vi "GUI_HTU_EMQ_triplet.vi"() -> ()   [LabVIEW 2020]
uses:
  Shared/GUI_Template/GUI_master/tcp_new_data_event.ctl
  Shared/GUI_Template/GUI_master/tcp new data cluster.ctl
panel:
  in  "abort3":bool
  in  "abort2":bool
  out "Chart":cluster{dbl, dbl, dbl}(graph)
  in  "Degauss max\ncurrent":dbl=1.0
  in  "EMQ3":bool
  in  "EMQ2":bool
  out "EMQ3 indicator":bool
  out "EMQ2 indicator":bool
  out "EMQ1 indicator":bool
  in  "EMQ1":bool
  in  "abort1":bool
  in  "SwitchWait":dbl=1500.0 min=0.0 max=12.0
  in  "EMQ3Reset":bool caption="Blank Button"
  in  "EMQ3Switch":bool caption="Blank Button"
  in  "EMQ2Reset":bool caption="Blank Button"
  in  "EMQ2Switch":bool caption="Blank Button"
  in  "EMQ1Reset":bool caption="Blank Button"
  in  "EMQ1Switch":bool caption="Blank Button"
  in  "DigitalOutput.Channel 4::4":bool=TRUE caption="Blank Button"
  in  "DigitalOutput.Channel 5::4":bool=TRUE caption="Blank Button"
  in  "DigitalOutput.Channel 2::4":bool=TRUE caption="Blank Button"
  in  "DigitalOutput.Channel 3::4":bool=TRUE caption="Blank Button"
  out "XY Graph":cluster{dbl[], dbl[]}(graph)
  in  "CurrentSwitch limit":dbl=0.03 min=0.0 max=12.0
  in  "GUIdevice 4":string="U_SSR_2"
  out "Power.Ch2::1":dbl caption="Power::2" min=0.0 max=12.0
  out "Voltage.Ch2::1":dbl caption="Voltage::2" min=0.0 max=12.0
  out "Current.Ch2::1":dbl caption="Current::2" min=0.0 max=12.0
  out "Power.Ch3::1":dbl caption="Power::3" min=0.0 max=12.0
  out "Voltage.Ch3::1":dbl caption="Voltage::3" min=0.0 max=12.0
  out "Current.Ch3::1":dbl caption="Current::3" min=0.0 max=12.0
  out "Power.Ch1::1":dbl caption="Power::1" min=0.0 max=12.0
  out "Voltage.Ch1::1":dbl caption="Voltage::1" min=0.0 max=12.0
  out "Current.Ch1::1":dbl caption="Current::1" min=0.0 max=12.0
  in  "Voltage_Limit.Ch3::1":dbl caption="EMQ3 Voltage" min=0.0 max=6.0
  in  "Enable_Output.Ch3::1":enum16{"on", "off"}(ring) caption="Enable EMQ3"
  in  "Current_Limit.Ch3::1":dbl caption="EMQ3 Current" min=0.0 max=6.0
  in  "Voltage_Limit.Ch1::1":dbl caption="EMQ1 Voltage" min=0.0 max=6.0
  in  "Voltage_Limit.Ch2::1":dbl caption="EMQ2 Voltage" min=0.0 max=8.0
  in  "Enable_Output.Ch2::1":enum16{"on", "off"}(ring) caption="Enable EMQ2"
  in  "Enable_Output.Ch1::1":enum16{"on", "off"}(ring) caption="Enable EMQ1"
  in  "Current_Limit.Ch1::1":dbl caption="EMQ1 Current" min=0.0 max=6.0
  in  "Current_Limit.Ch2::1":dbl caption="EMQ2 Current" min=0.0 max=6.0
  in  "UDP error message":string
  in  "GUIdevice 1":string="U_EMQTriplet"
  in  "DigitalOutput.Channel 0::4":bool=TRUE caption="Blank Button"
  in  "DigitalOutput.Channel 1::4":bool=TRUE caption="Blank Button"
  out "error IO 2":errorcluster
  out "tcp data event":T1
  in  "stop":bool
  # "HTU EMQ Triplet"
  # "Polarity indicator"
  # "Polarity switch"
  # "Polarity reset"
  # "Degaussing"
  # "EMQ1\nEMQ1"
  # "EMQ2\nEMQ2"
  # "EMQ3"
  # "Enable output"
  # "Current Limit"
  # "Voltage Limit"
  # "Current"
  # "Voltage"
  # "Power"
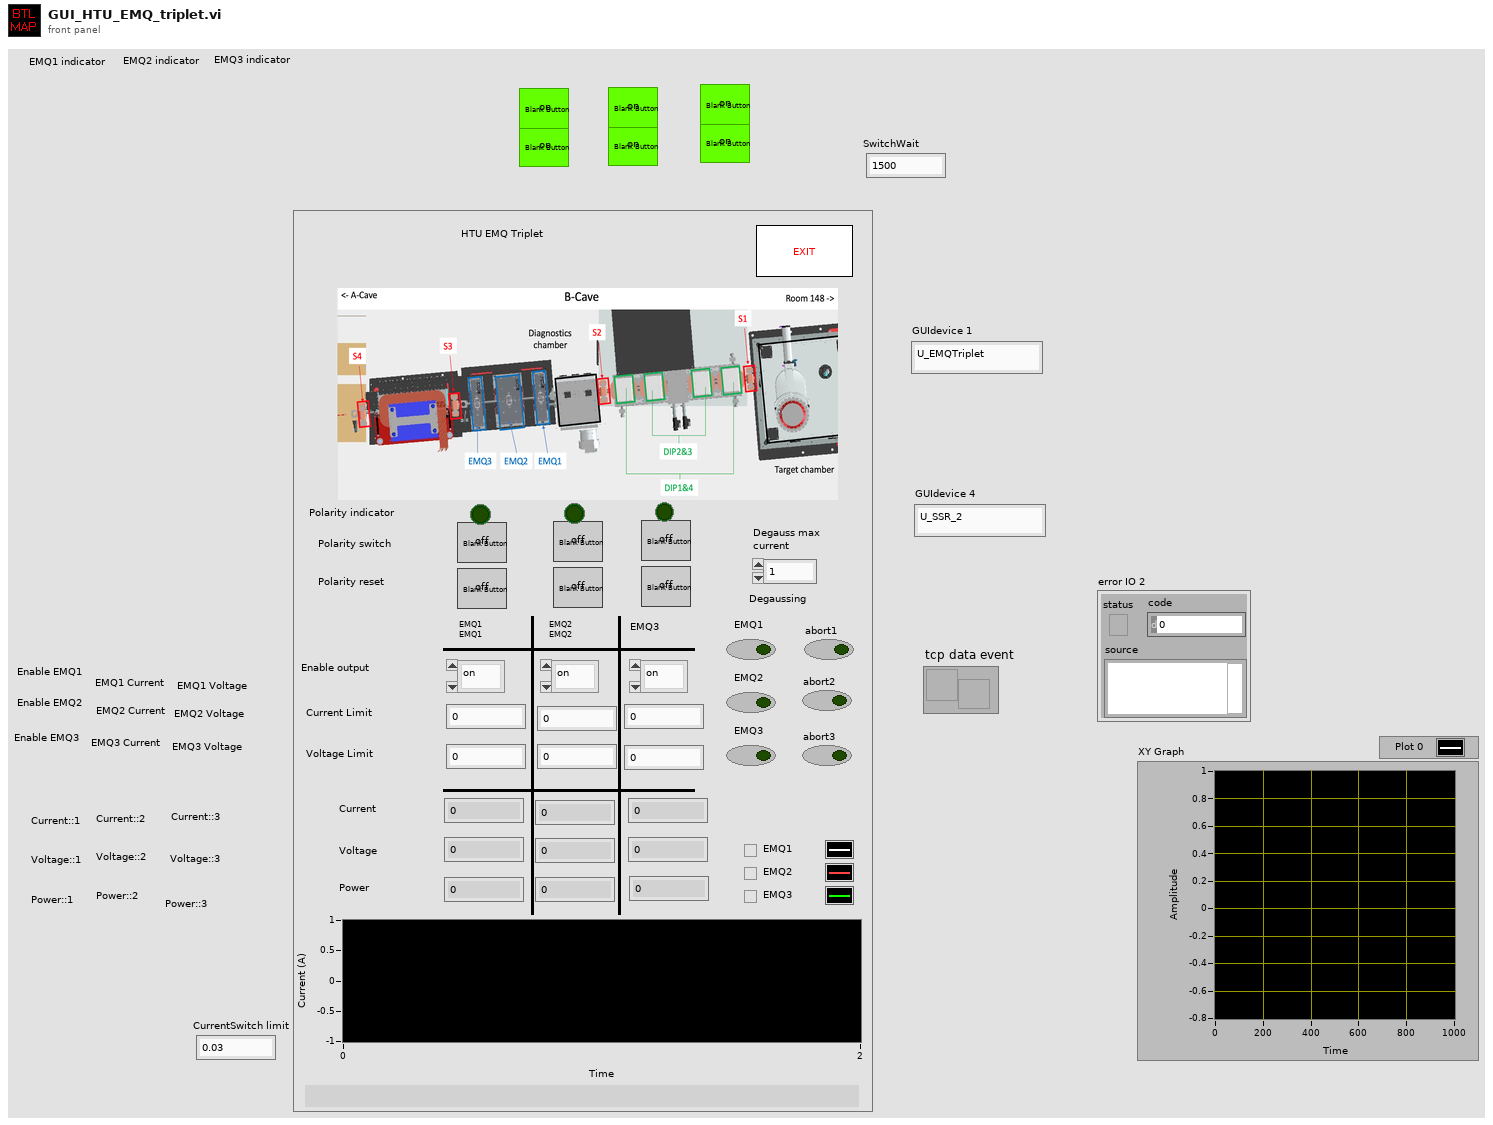
[diagram p1: front panel]
types:
  T1 = typedef "tcp_new_data_event.ctl" = refnum<user-event>
  T2 = typedef "tcp new data cluster.ctl" = cluster{"EventEnum":enum16{"new data", "connection status update"}, "Device name":string}
  T3 = enum32{"invalid app kind", "Development System", "Run Time System", "Student Edition", "Embedded LabVIEW", "Evaluation", "Custom"}
  T4 = enum32{"Invalid", "Standard", "Closed", "Hidden", "Minimized", "Maximized"}
  T5 = cluster{"Core":cluster{"Current VI Reference":refnum<vi>, "Close Panel on Exit?":bool}, "CurrentGraph1":dbl[][], "EMQ1PolaritySwitched":bool, "EMQ2PolaritySwitched":bool, "EMQ3PolaritySwitched":bool, "DegaussEMQ1":bool, "degauss loop":i32, "EMQ1DegaussSetCur":dbl, "EMQ2DegaussSetCur":dbl, "EMQ3DegaussSetCur":dbl, "last chart update tck":i32}
  T6 = cluster{"Current VI Reference":refnum<vi>, "Close Panel on Exit?":bool}
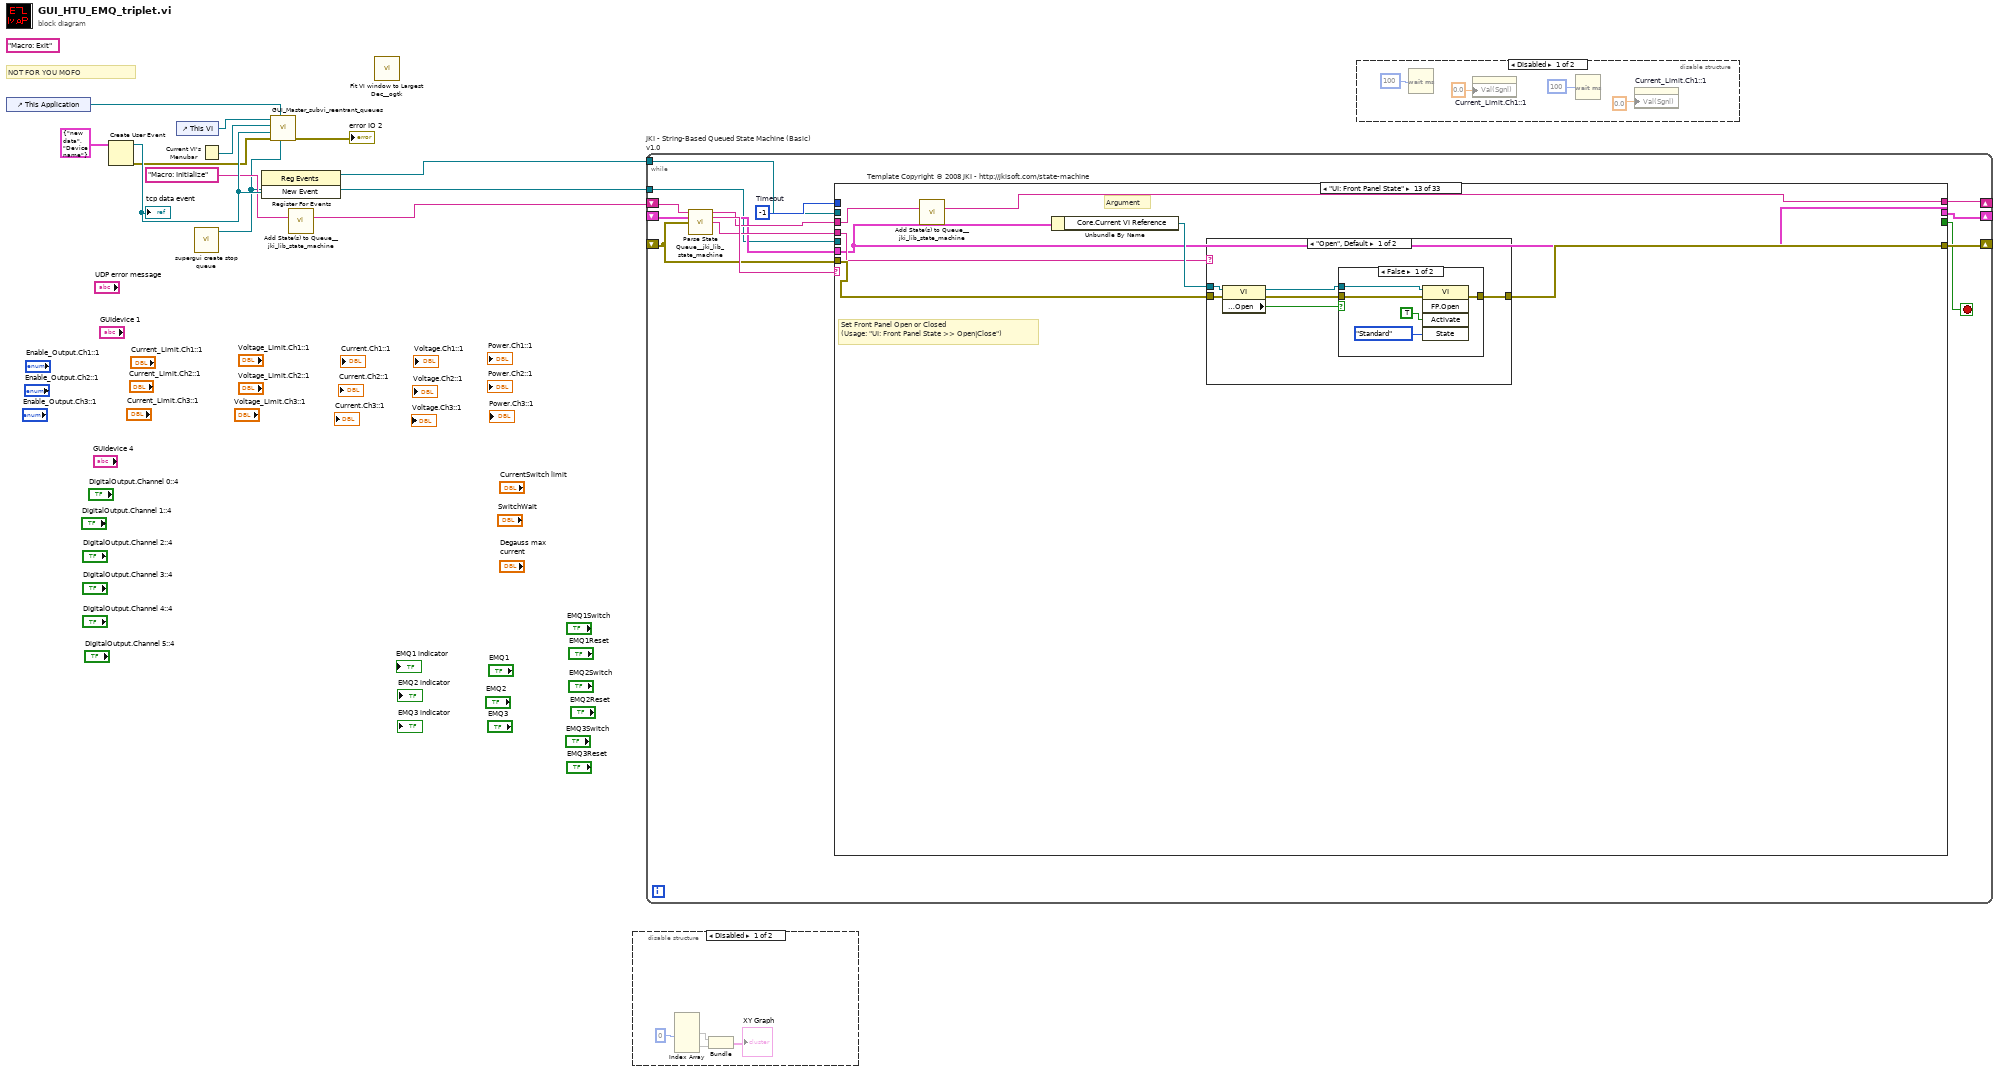
[diagram p0: block diagram]
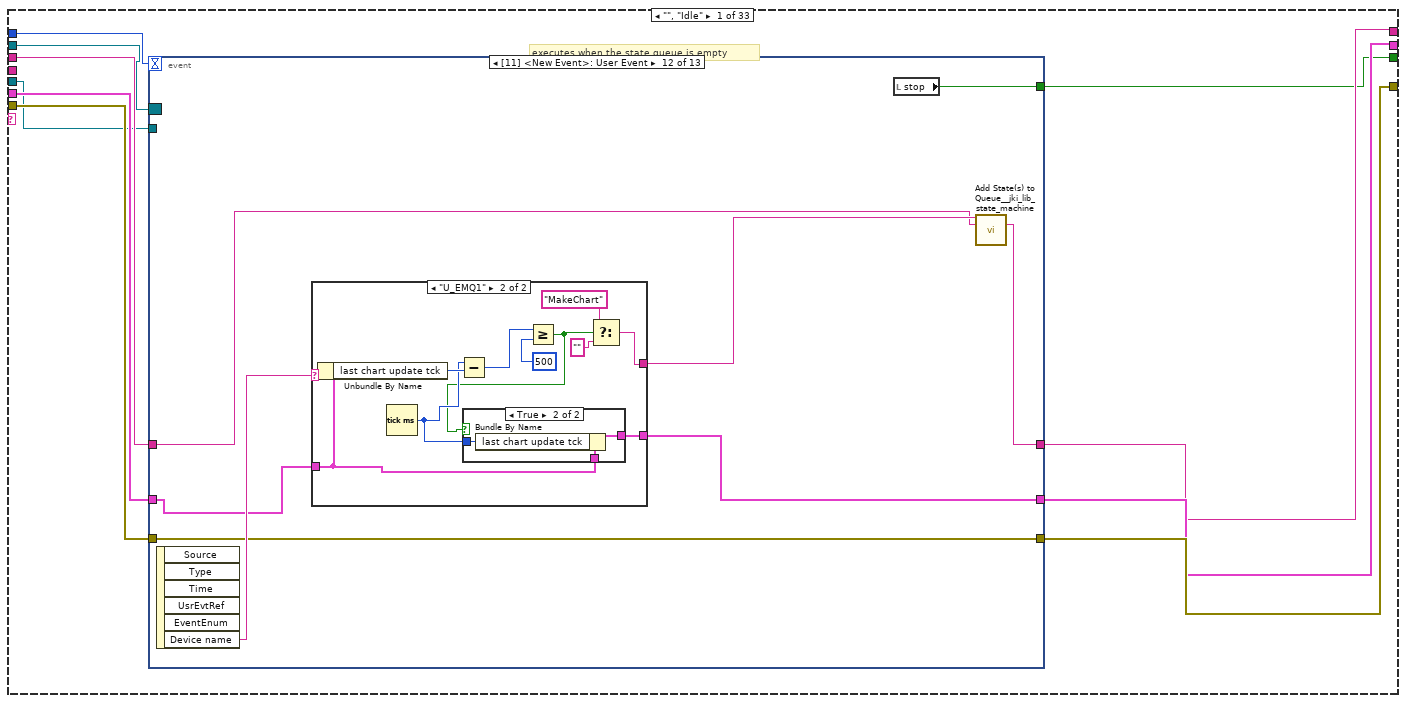
[diagram p4: hidden frame]
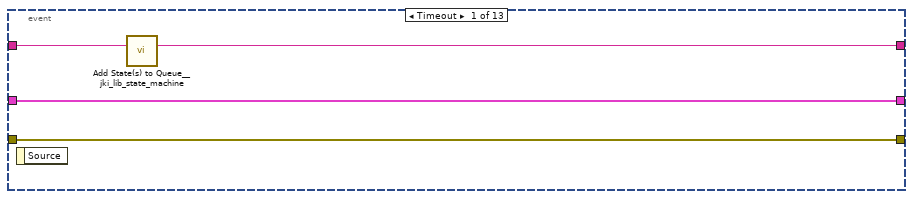
[diagram p5: hidden frame]
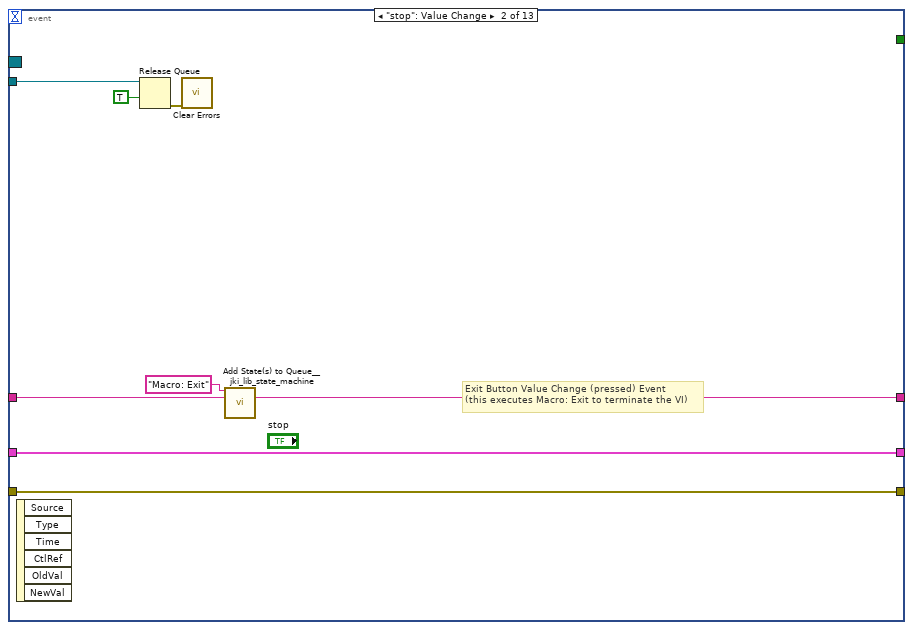
[diagram p6: hidden frame]
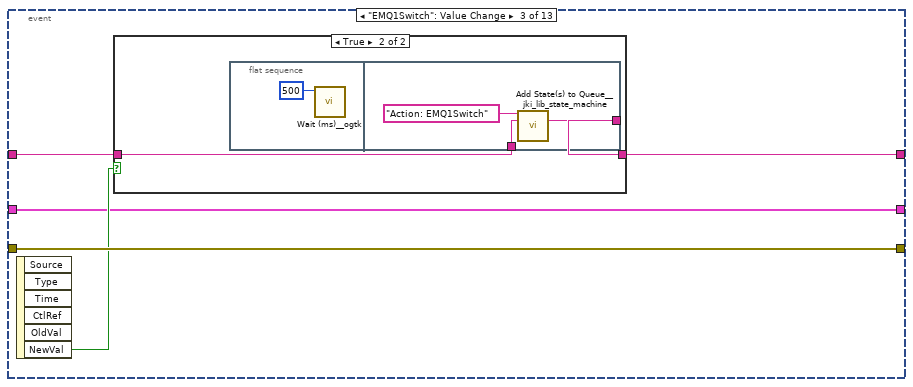
[diagram p7: hidden frame]
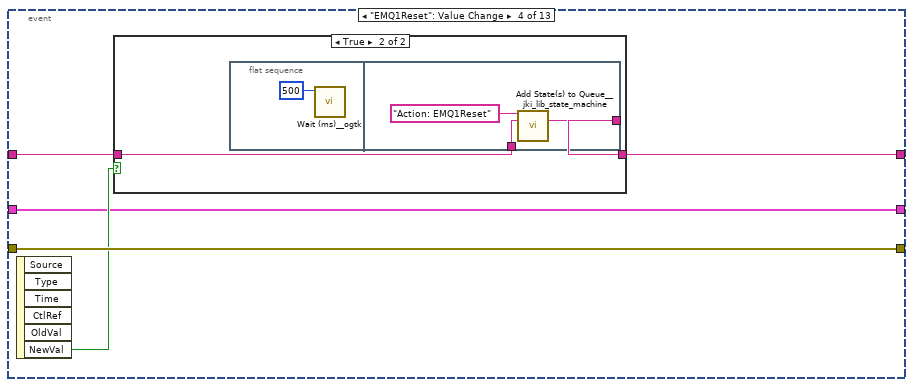
[diagram p9: hidden frame]
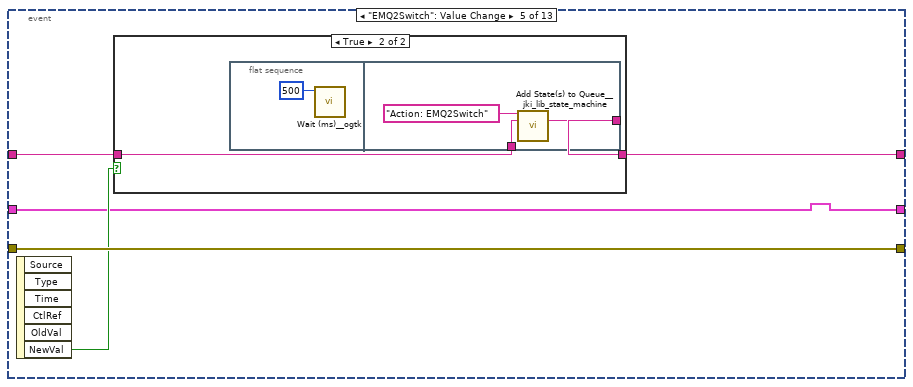
[diagram p11: hidden frame]
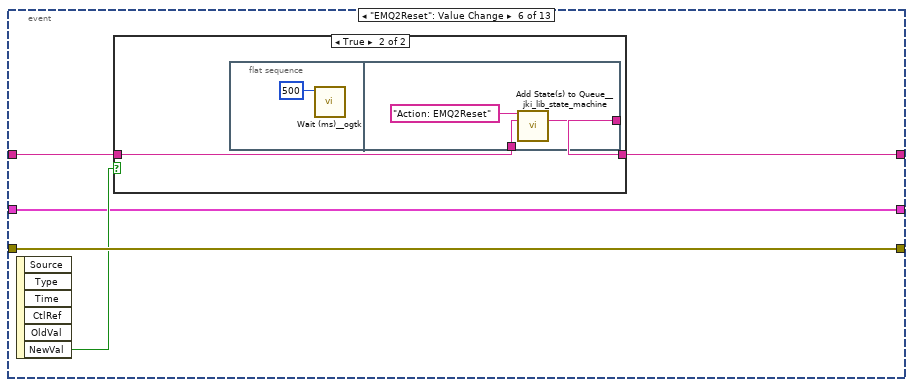
[diagram p13: hidden frame]
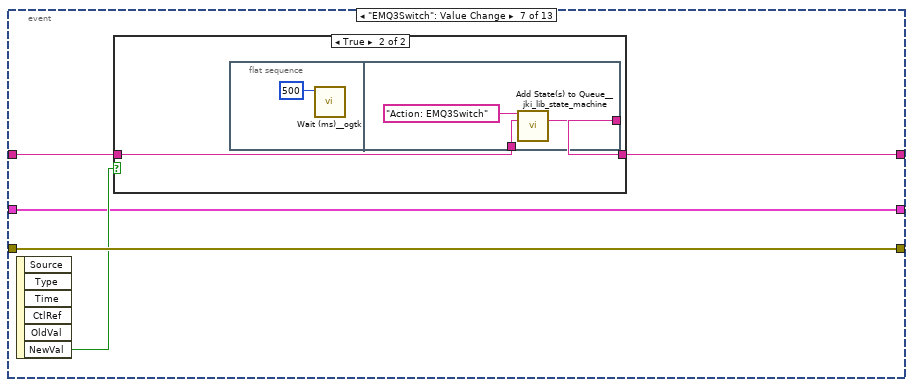
[diagram p15: hidden frame]
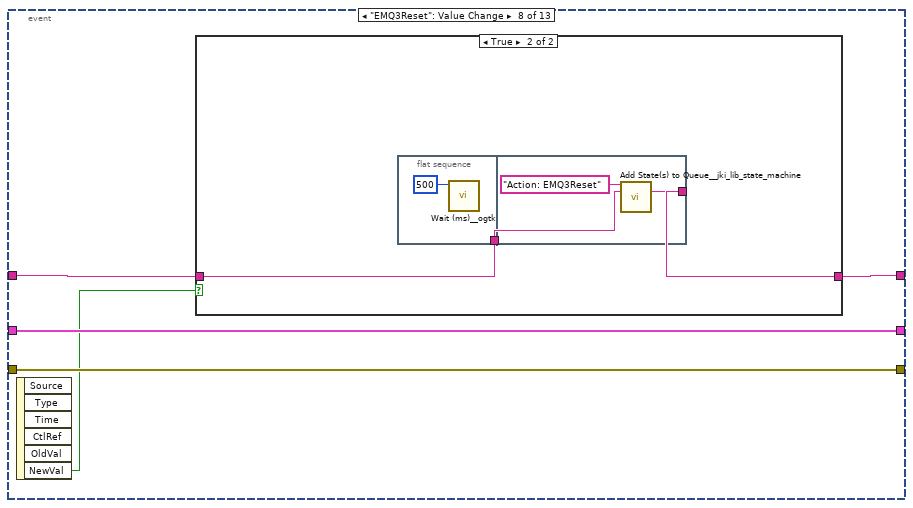
[diagram p17: hidden frame]
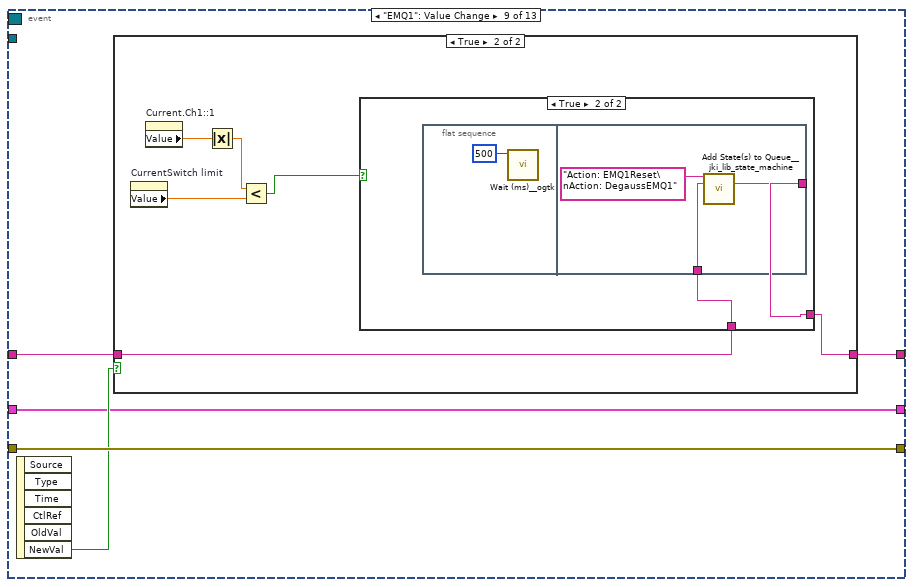
[diagram p19: hidden frame]
diagram:
  (unwired) "Macro: Exit"
  # "NOT FOR YOU MOFO"
  n1 = control-ref of="This Application"() -> (w11:refnum<vi>)
  n2 = Create User Event(user event datatype=T2 {"EventEnum"=enum."new data", "Device name"="Device name"} ("New Event")) -> (user event=w10:refnum<user-event>, error out=w9:errorcluster)  [unwired: 1 in]
  "tcp data event" <- w10
  n3 = control-ref of="This VI"() -> (w5:refnum<vi>)
  n4 = call "supergui create stop queue.vi"() -> ("STOP Queue out"=w1:refnum<queue>)  [unwired: 11 in]
  n5 = Current VI's Menubar() -> (w7:refnum<k9>)
  n6 = register-events(w10) -> (reference out=w2:refnum<event-registration>)  [unwired: 2 in, 1 out]
  n7 = call "GUI_Master_subvi_reentrant_queues.vi"("STOP Queue in"=w1, "This Application"=w11, "error in (no error)"=w9, "tcp data event"=w10, "Caller menu reference"=w7, "Caller VI ref"=w5) -> ("error out"=→"error IO 2":errorcluster)  [unwired: 5 in]
  n8 = call <vilib>:"Add State(s) to Queue__jki_lib_state_machine.vi"("State(s) in (\"\")"="Macro: Initialize") -> ("States Out"=w3:string)  [unwired: 14 in]
  n9 = call <userlib>:"Fit VI window to Largest Dec__ogtk.vi"() -> ()  [unwired: 6 in, 2 out]
  n10 = disable-structure shown="Disabled" {
    frame Disabled {
      n11 = Index Array(index (col) #1=0 ("disabled index (col)")) -> (array=w16:dbl[][], element #1=w12, element #2=w13)  [unwired: 3 in]
      n12 = Bundle(w12, w13) -> (→"XY Graph":cluster{void, void})  [unwired: 1 in]
    }
    frame Enabled {
    }
  }
  n13 = while "JKI - String-Based Queued State Machine (Basic) v1.0" {
    shift-right: [w23] -> _
    shift-left: _ -> [w22]
    shift-right: [w25] -> _
    shift-left: _ -> [w20]
    shift-right: [w17] -> _
    shift-left: w3 -> [w26]
    tunnel: w2 -> [w19]
    tunnel: w1 -> [w18]
    stop <- w24 stop-if-true
    w21 = -1  # Timeout
    # "Template Copyright © 2008 JKI - http://jkisoft.com/state-machine"
    n14 = call <vilib>:"Parse State Queue__jki_lib_state_machine.vi"("State Queue"=w26, "Error In (no error)"=w20) -> ("Remaining States"=w28:string, "Current State"=w29:string, "Arguments"=w27:string)  [unwired: 11 in]
    n15 = case shown="\"UI: Front Panel State\"" w29 {
      selector: w29 -> [_ _ w215 _ _ _ _ _ _ _ _ _ _ _ _ _ _ _ _ _ _ _ _ _ _ _ _ _ _ _ _ _ _]
      tunnel: w28 -> [w39 w213 w218 w236 w242 w247 w251 w266 w272 w276 w280 w286 w297 w323 w328 w338 w342 w352 w375 w398 w421 w444 w467 w486 w496 w506 w517 w585 w653 w716 w733 w749 w777]
      tunnel: w27 -> [_ _ _ _ _ _ _ _ _ _ _ w282 w293 _ _ _ _ _ _ _ _ _ _ _ _ _ _ _ _ _ _ _ _]
      tunnel: w22 -> [w38 w211 w217 w228 w241 w246 w249 _ w268 w274 w279 w285 w292 w321 w326 w330 w340 w346 w369 w392 w415 w436 w459 w484 w494 w504 w518 w586 w654 w720 w736 w752 w767]
      tunnel: [w37 w212 w220 w225 errorcluster {"status"=FALSE, "code"=0, "source"=""} ("error out") w245 w250 w265 w270 w275 w278 w283 w295 w322 w327 w337 w341 w343 w366 w389 w412 w437 w460 w487 w497 w507 w511 w579 w647 w721 w737 w753 w778] -> w25
      tunnel: w20 -> [w36 w212 w219 w225 w240 w245 w250 w265 w271 w275 w278 w284 w296 w322 w327 w337 w341 w344 w367 w390 w413 w438 w461 w487 w497 w507 w512 w580 w648 w721 w737 w753 w778]
      tunnel: [w30 _ _ _ _ TRUE _ _ _ _ _ _ _ _ _ _ _ _ _ _ _ _ _ _ _ _ _ _ _ _ _ _ _] -> w24
      tunnel: [w33 w211 w217 w227 w241 w246 w249 w255 w268 w274 w279 w285 w292 w321 w326 w330 w340 w345 w368 w391 w414 w435 w458 w483 w493 w503 w515 w583 w651 w720 w736 w752 w767] -> w23
      tunnel: w21 -> [w35 _ _ _ _ _ _ _ _ _ _ _ _ _ _ _ _ _ _ _ _ _ _ _ _ _ _ _ _ _ _ _ _]
      tunnel: w19 -> [w31 _ _ _ _ _ _ _ _ _ _ _ _ _ _ _ _ _ _ _ _ _ _ _ _ _ _ _ _ _ _ _ _]
      tunnel: w18 -> [w34 _ _ _ _ _ _ _ _ _ _ _ _ _ _ _ _ _ _ _ _ _ _ _ _ _ _ _ _ _ _ _ _]
      tunnel: [w32 w210 w214 w226 w237 w243 w248 w261 w267 w273 w277 w281 w291 w320 w324 w329 w339 w351 w374 w397 w420 w443 w466 w485 w495 w505 w516 w584 w652 w718 w734 w750 w777] -> w17
      frame "", "Idle" {
        # "executes when the state queue is empty"
        n16 = event shown="[11] <New Event>: User Event" {
          selector: w31 -> [_ _ _ _ _ _ _ _ _ _ _ _ _]
          dyn-events: _ -> [_ _ _ _ _ _ _ _ _ _ _ _ _]
          timeout: w35 -> [_ _ _ _ _ _ _ _ _ _ _ _ _]
          tunnel: w39 -> [w43 w51 w54 w66 w78 w90 w102 w115 w126 w145 w164 w186 w209]
          tunnel: [w42 w50 w53 w65 w77 w89 w101 w114 w125 w144 w163 w185 w208] -> w32
          tunnel: w38 -> [w40 w48 w52 w64 w76 w88 w100 w113 w124 w143 w162 w182 w206]
          tunnel: [w41 w49 w56 w68 w80 w92 w104 w116 w128 w147 w166 w184 w207] -> w37
          tunnel: w36 -> [w41 w49 w56 w68 w80 w92 w104 w116 w128 w147 w166 w184 w207]
          tunnel: [w40 w48 w52 w64 w76 w88 w100 w113 w124 w143 w162 w181 w206] -> w33
          tunnel: w34 -> [_ w45 _ _ _ _ _ _ _ _ _ _ _]
          tunnel: [_ _ _ _ _ _ _ _ _ _ _ w183 _] -> w30
          event Timeout {
            n17 = event-data() -> ()  [unwired: 1 in, 1 out]
            n18 = call <vilib>:"Add State(s) to Queue__jki_lib_state_machine.vi"("State(s) in (\"\")"=w43) -> ("States Out"=w42:string)  [unwired: 14 in]
          }
          event "stop": Value Change {
            # "Exit Button Value Change (pressed) Event\n(this executes Macro: Exit to terminate the VI)"
            n19 = event-data() -> ()  [unwired: 1 in, 6 out]
            n20 = Release Queue(queue=w45, force destroy? (F)=TRUE) -> (error out=w46:errorcluster)  [unwired: 1 in, 2 out]
            n21 = call <vilib>:"Clear Errors.vi"("error in (no error)"=w46) -> ()  [unwired: 5 in, 2 out]
            n22 = call <vilib>:"Add State(s) to Queue__jki_lib_state_machine.vi"("State(s) in Front (\"\")"="Macro: Exit", "State(s) in (\"\")"=w51) -> ("States Out"=w50:string)  [unwired: 13 in]
          }
          event "EMQ1Switch": Value Change {
            n23 = event-data() -> ("NewVal"=w55:bool)  [unwired: 1 in, 5 out]
            n24 = case shown="True" w55 {
              tunnel: w54 -> [w57 w59]
              tunnel: [w57 w58] -> w53
              frame False {
              }
              frame True {
                n25 = flat-sequence {
                  tunnel: w59 -> [w62]
                  tunnel: [w61] -> w58
                  frame #0 {
                    n26 = call <userlib>:"Wait (ms)__ogtk.vi"("milliseconds to wait"=u32 500) -> ()  [unwired: 9 in, 2 out]
                  }
                  frame #1 {
                    n27 = call <vilib>:"Add State(s) to Queue__jki_lib_state_machine.vi"("State(s) in Front (\"\")"="Action: EMQ1Switch" ("State(s) in Front (\"\")"), "State(s) in (\"\")"=w62) -> ("States Out"=w61:string)  [unwired: 13 in]
                  }
                }
              }
            }
          }
          event "EMQ1Reset": Value Change {
            n28 = event-data() -> ("NewVal"=w67:bool)  [unwired: 1 in, 5 out]
            n29 = case shown="True" w67 {
              tunnel: w66 -> [w69 w71]
              tunnel: [w69 w70] -> w65
              frame False {
              }
              frame True {
                n30 = flat-sequence {
                  tunnel: w71 -> [w74]
                  tunnel: [w73] -> w70
                  frame #0 {
                    n31 = call <userlib>:"Wait (ms)__ogtk.vi"("milliseconds to wait"=u32 500) -> ()  [unwired: 9 in, 2 out]
                  }
                  frame #1 {
                    n32 = call <vilib>:"Add State(s) to Queue__jki_lib_state_machine.vi"("State(s) in Front (\"\")"="Action: EMQ1Reset" ("State(s) in Front (\"\")"), "State(s) in (\"\")"=w74) -> ("States Out"=w73:string)  [unwired: 13 in]
                  }
                }
              }
            }
          }
          event "EMQ2Switch": Value Change {
            n33 = event-data() -> ("NewVal"=w79:bool)  [unwired: 1 in, 5 out]
            n34 = case shown="True" w79 {
              tunnel: w78 -> [w81 w83]
              tunnel: [w81 w82] -> w77
              frame False {
              }
              frame True {
                n35 = flat-sequence {
                  tunnel: w83 -> [w86]
                  tunnel: [w85] -> w82
                  frame #0 {
                    n36 = call <userlib>:"Wait (ms)__ogtk.vi"("milliseconds to wait"=u32 500) -> ()  [unwired: 9 in, 2 out]
                  }
                  frame #1 {
                    n37 = call <vilib>:"Add State(s) to Queue__jki_lib_state_machine.vi"("State(s) in Front (\"\")"="Action: EMQ2Switch" ("State(s) in Front (\"\")"), "State(s) in (\"\")"=w86) -> ("States Out"=w85:string)  [unwired: 13 in]
                  }
                }
              }
            }
          }
          event "EMQ2Reset": Value Change {
            n38 = event-data() -> ("NewVal"=w91:bool)  [unwired: 1 in, 5 out]
            n39 = case shown="True" w91 {
              tunnel: w90 -> [w93 w95]
              tunnel: [w93 w94] -> w89
              frame False {
              }
              frame True {
                n40 = flat-sequence {
                  tunnel: w95 -> [w98]
                  tunnel: [w97] -> w94
                  frame #0 {
                    n41 = call <userlib>:"Wait (ms)__ogtk.vi"("milliseconds to wait"=u32 500) -> ()  [unwired: 9 in, 2 out]
                  }
                  frame #1 {
                    n42 = call <vilib>:"Add State(s) to Queue__jki_lib_state_machine.vi"("State(s) in Front (\"\")"="Action: EMQ2Reset" ("State(s) in Front (\"\")"), "State(s) in (\"\")"=w98) -> ("States Out"=w97:string)  [unwired: 13 in]
                  }
                }
              }
            }
          }
          event "EMQ3Switch": Value Change {
            n43 = event-data() -> ("NewVal"=w103:bool)  [unwired: 1 in, 5 out]
            n44 = case shown="True" w103 {
              tunnel: w102 -> [w105 w107]
              tunnel: [w105 w106] -> w101
              frame False {
              }
              frame True {
                n45 = flat-sequence {
                  tunnel: w107 -> [w110]
                  tunnel: [w109] -> w106
                  frame #0 {
                    n46 = call <userlib>:"Wait (ms)__ogtk.vi"("milliseconds to wait"=u32 500) -> ()  [unwired: 9 in, 2 out]
                  }
                  frame #1 {
                    n47 = call <vilib>:"Add State(s) to Queue__jki_lib_state_machine.vi"("State(s) in Front (\"\")"="Action: EMQ3Switch" ("State(s) in Front (\"\")"), "State(s) in (\"\")"=w110) -> ("States Out"=w109:string)  [unwired: 13 in]
                  }
                }
              }
            }
          }
          event "EMQ3Reset": Value Change {
            n48 = event-data() -> ("NewVal"=w112:bool)  [unwired: 1 in, 5 out]
            n49 = case shown="True" w112 {
              tunnel: w115 -> [w117 w119]
              tunnel: [w117 w118] -> w114
              frame False {
              }
              frame True {
                n50 = flat-sequence {
                  tunnel: w119 -> [w122]
                  tunnel: [w121] -> w118
                  frame #0 {
                    n51 = call <userlib>:"Wait (ms)__ogtk.vi"("milliseconds to wait"=u32 500) -> ()  [unwired: 9 in, 2 out]
                  }
                  frame #1 {
                    n52 = call <vilib>:"Add State(s) to Queue__jki_lib_state_machine.vi"("State(s) in Front (\"\")"="Action: EMQ3Reset" ("State(s) in Front (\"\")"), "State(s) in (\"\")"=w122) -> ("States Out"=w121:string)  [unwired: 13 in]
                  }
                }
              }
            }
          }
          event "EMQ1": Value Change {
            n53 = event-data() -> ("NewVal"=w127:bool)  [unwired: 1 in, 5 out]
            n54 = case shown="True" w127 {
              tunnel: w126 -> [w129 w135]
              tunnel: [w129 w134] -> w125
              frame False {
              }
              frame True {
                n55 = property on="CurrentSwitch limit" class="DigNum (strict)"() -> ("Value"=w131:dbl)  [unwired: 2 in, 2 out]
                n56 = property on="Current.Ch1::1" class="DigNum (strict)"() -> ("Value"=w132:dbl)  [unwired: 2 in, 2 out]
                n57 = Absolute Value(x=w132) -> (abs(x)=w133:dbl)
                n58 = Less?(x=w133, y=w131) -> (x < y?=w130:bool)
                n59 = case shown="True" w130 {
                  tunnel: w135 -> [w136 w138]
                  tunnel: [w136 w137] -> w134
                  frame False {
                  }
                  frame True {
                    n60 = flat-sequence {
                      tunnel: w138 -> [w141]
                      tunnel: [w140] -> w137
                      frame #0 {
                        n61 = call <userlib>:"Wait (ms)__ogtk.vi"("milliseconds to wait"=u32 500) -> ()  [unwired: 9 in, 2 out]
                      }
                      frame #1 {
                        n62 = call <vilib>:"Add State(s) to Queue__jki_lib_state_machine.vi"("State(s) in Front (\"\")"="Action: EMQ1Reset\nAction: DegaussEMQ1" ("State(s) in Front (\"\")"), "State(s) in (\"\")"=w141) -> ("States Out"=w140:string)  [unwired: 13 in]
                      }
                    }
                  }
                }
              }
            }
          }
          event "EMQ2": Value Change {
            n63 = event-data() -> ("NewVal"=w146:bool)  [unwired: 1 in, 5 out]
            n64 = case shown="True" w146 {
              tunnel: w145 -> [w148 w154]
              tunnel: [w148 w153] -> w144
              frame False {
              }
              frame True {
                n65 = property on="CurrentSwitch limit" class="DigNum (strict)"() -> ("Value"=w150:dbl)  [unwired: 2 in, 2 out]
                n66 = property on="Current.Ch2::1" class="DigNum (strict)"() -> ("Value"=w151:dbl)  [unwired: 2 in, 2 out]
                n67 = Absolute Value(x=w151) -> (abs(x)=w152:dbl)
                n68 = Less?(x=w152, y=w150) -> (x < y?=w149:bool)
                n69 = case shown="True" w149 {
                  tunnel: w154 -> [w155 w157]
                  tunnel: [w155 w156] -> w153
                  frame False {
                  }
                  frame True {
                    n70 = flat-sequence {
                      tunnel: w157 -> [w160]
                      tunnel: [w159] -> w156
                      frame #0 {
                        n71 = call <userlib>:"Wait (ms)__ogtk.vi"("milliseconds to wait"=u32 500) -> ()  [unwired: 9 in, 2 out]
                      }
                      frame #1 {
                        n72 = call <vilib>:"Add State(s) to Queue__jki_lib_state_machine.vi"("State(s) in Front (\"\")"="Action: EMQ2Reset\nAction: DegaussEMQ2" ("State(s) in Front (\"\")"), "State(s) in (\"\")"=w160) -> ("States Out"=w159:string)  [unwired: 13 in]
                      }
                    }
                  }
                }
              }
            }
          }
          event "EMQ3": Value Change {
            n73 = event-data() -> ("NewVal"=w165:bool)  [unwired: 1 in, 5 out]
            n74 = case shown="True" w165 {
              tunnel: w164 -> [w167 w173]
              tunnel: [w167 w172] -> w163
              frame False {
              }
              frame True {
                n75 = property on="CurrentSwitch limit" class="DigNum (strict)"() -> ("Value"=w169:dbl)  [unwired: 2 in, 2 out]
                n76 = property on="Current.Ch3::1" class="DigNum (strict)"() -> ("Value"=w170:dbl)  [unwired: 2 in, 2 out]
                n77 = Absolute Value(x=w170) -> (abs(x)=w171:dbl)
                n78 = Less?(x=w171, y=w169) -> (x < y?=w168:bool)
                n79 = case shown="True" w168 {
                  tunnel: w173 -> [w174 w176]
                  tunnel: [w174 w175] -> w172
                  frame False {
                  }
                  frame True {
                    n80 = flat-sequence {
                      tunnel: w176 -> [w179]
                      tunnel: [w178] -> w175
                      frame #0 {
                        n81 = call <userlib>:"Wait (ms)__ogtk.vi"("milliseconds to wait"=u32 500) -> ()  [unwired: 9 in, 2 out]
                      }
                      frame #1 {
                        n82 = call <vilib>:"Add State(s) to Queue__jki_lib_state_machine.vi"("State(s) in Front (\"\")"="Action: EMQ3Reset\nAction: DegaussEMQ3" ("State(s) in Front (\"\")"), "State(s) in (\"\")"=w179) -> ("States Out"=w178:string)  [unwired: 13 in]
                      }
                    }
                  }
                }
              }
            }
          }
          event User Event {
            n83 = event-data() -> ("Device name"=w187:string)  [unwired: 1 in, 5 out]
            n84 = case shown="\"U_EMQ1\"" w187 {
              tunnel: [_ w192] -> w188
              tunnel: w182 -> [w189 w198]
              tunnel: [w189 w199] -> w181
              frame "False", Default {
              }
              frame "U_EMQ1" {
                n85 = Unbundle By Name(w198) -> ("last chart update tck"=w197:i32)
                n86 = Tick Count (ms)() -> (millisecond timer value=w191:u32)
                n87 = Subtract(x=w191, y=w197) -> (x-y=w196:u32)
                n88 = Greater Or Equal?(x=w196, y=u32 500 ("x")) -> (x >= y?=w190:bool)
                n89 = case shown="True" w190 {
                  tunnel: [w200 w203] -> w199
                  tunnel: w198 -> [w200 w202]
                  tunnel: w191 -> [_ w201]
                  frame False {
                  }
                  frame True {
                    n90 = Bundle By Name(cluster=w202, "last chart update tck"=w201) -> (w203:T5)
                  }
                }
                n91 = Select(t="MakeChart", s=w190, f="") -> (s? t:f=w192:string)
              }
            }
            n92 = local read "stop"() -> (w183:bool)
            n93 = call <vilib>:"Add State(s) to Queue__jki_lib_state_machine.vi"("State(s) in Front (\"\")"=w188, "State(s) in (\"\")"=w186) -> ("States Out"=w185:string)  [unwired: 13 in]
          }
          event Panel Close? {
            # "Discard the event because we'll close the front panel ourselves in Macro: Exit"
            # "Close Panel button (pressed) Event\n(this executes Macro: Exit to terminate the VI)"
            n94 = event-data() -> ()  [unwired: 1 in, 1 out]
            n95 = call <vilib>:"Add State(s) to Queue__jki_lib_state_machine.vi"("State(s) in Front (\"\")"="Macro: Exit", "State(s) in (\"\")"=w209) -> ("States Out"=w208:string)  [unwired: 13 in]
            n96 = event-data("Discard?"=TRUE) -> ()  [unwired: 1 in, 1 out]
          }
        }
      }
      frame "---------- Core ----------" {
        # "Do not put any code in this frame.\n(it is a separator no-op)"
        n97 = call <vilib>:"Add State(s) to Queue__jki_lib_state_machine.vi"("State(s) in (\"\")"=w213) -> ("States Out"=w210:string)  [unwired: 14 in]
      }
      frame Default {
        w223 = 42 items=["No error", "Argument error", "Memory is full", "Out of zone", "End of file", "File already open", "Generic file I/O error", "File not found", "File permission error", "Disk is full", "Duplicate path", "Too many files open", "System feature not enabled", "Resource file not found", "Cannot add resource", "Resource not found", "Image not found", "Image memory error", "Pen does not exist", "Config type invalid", "Config token not found", "Config parse error", "Config memory error", "Bad external code format", "Bad external code offset", "External code not present", "Null window", "Destroy window error", "Null menu", "Print aborted", "Bad print record", "Print driver error", "Windows error during printing", "Memory error during printing", "Print dialog error", "Generic print error", "Invalid device refnum", "Device not found", "Device parameter error", "Device unit error", "Cannot open device", "Device call aborted", "Generic error", "Cancelled by user", "Object ID too low", "Object ID too high", "Object not in heap", "Unknown heap", "Unknown object (invalid DefProc)", "Unknown object (DefProc not in table)", "Message out of range", "Invalid (null) method", "Unknown message", "Manager call not supported", "Bad address", "Network operation in progress", "Network operation timed out", "Connection is busy", "Network attribute not supported", "Network error", "Address in use", "System out of memory", "Connection aborted", "Connection refused", "Not connected", "Already connected", "Connection closed", "Initialization error (interapplication manager)", "Bad occurrence", "Wait on unbound occurrence handler", "Occurrence queue overflow", "Datalog type conflict", "Unused", "Unrecognized type (interapplication manager)", "Memory corrupt", "Failed to make temporary DLL", "Old CIN version", "Drag socket not found", "Failed to load drop-object", "Failed to register OLE object", "Failed to release OLE object", "Format specifier type mismatch", "Unknown format specifier", "Too few format specifiers", "Too many format specifiers", "Scan failed", "Newer CIN version", "Error converting to variant", "Runtime menu error", "Password tampered", "Variant attribute not found", "Incompatible variant data type", "Event data is not available", "Event Store is not present", "Occurrence is not found", "Event Queue is not created", "Event info is not available", "Refnum passed is NULL", "Error retrieving Class GUID", "Error retrieving CoClass GUID", "Error retrieving TypeLib GUID.", "Bad built application magic bytes.", "Specific driver is different from the specific driver associated with the Logical Name.", "There is no session opened to the class driver.", "Max Error", "MAX - Error with config objects", "MAX - Error loading configuration", "MAX - Group not supported"]
        # "Current State"
        # "Do not delete, rename, or modify this frame.\n(this is used to capture unhandled states and typos)"
        # "Handle mistyped state name (developer tool)"
        n98 = call <vilib>:"Add State(s) to Queue__jki_lib_state_machine.vi"("State(s) in (\"\")"=w218) -> ("States Out"=w214:string)  [unwired: 14 in]
        n99 = Format Into String(format string="Software Exception: Unhandled State \"%s\"." ("message"), error in=w219, w215) -> (resulting string=w222:string, error out=w221:errorcluster)  [unwired: 1 in]
        n100 = call <vilib>:"Error Cluster From Error Code.vi"("show call chain? (False)"=TRUE, "error in (no error)"=w221, "error message (\"\")"=w222, "error code (0)"=w223) -> ("error out"=w220:errorcluster)  [unwired: 5 in]
      }
      frame "Initialize Core Data" {
        # "Do not delete, rename, or modify this frame.\n(this is used to determine panel behavior on exit)"
        # "originally closed?"
        # "exe?"
        # "If panel starts closed or is an EXE, then close it when we exit"
        n101 = call <vilib>:"Add State(s) to Queue__jki_lib_state_machine.vi"("State(s) in (\"\")"=w236) -> ("States Out"=w226:string)  [unwired: 14 in]
        n102 = property class="App"() -> ("App.Kind"=w234:T3)  [unwired: 2 in, 2 out]
        n103 = property class="VI"() -> ("Front Panel.Open"=w235:bool)  [unwired: 2 in, 2 out]
        n104 = Equal?(x=w234, y=T3."Run Time System" ("Application:Kind")) -> (x = y?=w231:bool)
        n105 = Not(x=w235) -> (.not. x?=w232:bool)
        n106 = Or(x=w232, y=w231) -> (x .or. y?=w230:bool)
        n107 = control-ref of="Current VI Reference"() -> (w229:refnum<vi>)
        n108 = Bundle By Name(cluster=w228, "Core.Current VI Reference"=w229, "Core.Close Panel on Exit?"=w230) -> (w227:T5)
      }
      frame "Error Handler" {
        # "Unhandled Error -- Display it"
        # "Handle any errors here.\nYou can also output any states to clean-up after errors occur"
        # "Clear error"
        n109 = call <vilib>:"General Error Handler.vi"("error in (no error)"=w240) -> ()  [unwired: 10 in, 5 out]
        n110 = call <vilib>:"Add State(s) to Queue__jki_lib_state_machine.vi"("State(s) in Front (\"\")"="/* Post Error States", "State(s) in (\"\")"=w242) -> ("States Out"=w237:string)  [unwired: 13 in]
      }
      frame "Exit" {
        # "Do not put any code in this frame.\n(No errors that occur here will be handled.)"
        n111 = call <vilib>:"Add State(s) to Queue__jki_lib_state_machine.vi"("State(s) in (\"\")"=w247) -> ("States Out"=w243:string)  [unwired: 14 in]
      }
      frame "---------- Data ----------" {
        # "Do not put any code in this frame.\n(It is a separator no-op. You can make a copy of this frame to create a new Data frame)"
        n112 = call <vilib>:"Add State(s) to Queue__jki_lib_state_machine.vi"("State(s) in (\"\")"=w251) -> ("States Out"=w248:string)  [unwired: 14 in]
      }
      frame "Data: Initialize" {
        w252 = 0  # last chart update tck
        w253 = 0.0  # EMQ3DegaussSetCur
        w254 = 0.0  # EMQ2DegaussSetCur
        w256 = 0.0  # EMQ1DegaussSetCur
        w257 = 0  # degauss loop
        w258 = FALSE  # DegaussEMQ1
        w259 = FALSE  # EMQ3PolaritySwitched
        w260 = FALSE  # EMQ2PolaritySwitched
        w262 = FALSE  # EMQ1PolaritySwitched
        w263 = dbl[][] []  # CurrentGraph1
        w264 = T6 {"Current VI Reference"=refnum, "Close Panel on Exit?"=FALSE}  # Core
        # "do not delete - used by framework"
        # "Initialize the shift-register data, here.\n(data names are defined by what you wire into the bundle function)"
        n113 = Bundle("Core"=w264, "CurrentGraph1"=w263, "EMQ1PolaritySwitched"=w262, "EMQ2PolaritySwitched"=w260, "EMQ3PolaritySwitched"=w259, "DegaussEMQ1"=w258, "degauss loop"=w257, "EMQ1DegaussSetCur"=w256, "EMQ2DegaussSetCur"=w254, "EMQ3DegaussSetCur"=w253, "last chart update tck"=w252) -> (w255:T5)  [unwired: 1 in]
        n114 = call <vilib>:"Add State(s) to Queue__jki_lib_state_machine.vi"("State(s) in (\"\")"=w266) -> ("States Out"=w261:string)  [unwired: 14 in]
      }
      frame "Data: Cleanup" {
        # "Cleanup any data and references, here.\n(this is called automatically, by the Macro: Exit)"
        n115 = call <vilib>:"Add State(s) to Queue__jki_lib_state_machine.vi"("State(s) in (\"\")"=w272) -> ("States Out"=w267:string)  [unwired: 14 in]
        n116 = Unbundle By Name(w268) -> ("Core.Current VI Reference"=w269:refnum<vi>)
        n117 = Close Reference(reference=w269, error in (no error)=w271) -> (error out=w270:errorcluster)
      }
      frame "---------- UI ----------" {
        # "Do not put any code in this frame.\n(It is a separator no-op. You can make a copy of this frame to create a new UI frame)"
        n118 = call <vilib>:"Add State(s) to Queue__jki_lib_state_machine.vi"("State(s) in (\"\")"=w276) -> ("States Out"=w273:string)  [unwired: 14 in]
      }
      frame "UI: Initialize" {
        # "Initialize the User Interface, here.\n(this is called automatically, by the Macro: Init)"
        n119 = call <vilib>:"Add State(s) to Queue__jki_lib_state_machine.vi"("State(s) in (\"\")"=w280) -> ("States Out"=w277:string)  [unwired: 14 in]
      }
      frame "UI: Cursor Set" {
        # "Argument"
        # "Set and Unset Cursor Busy.\n(Usage: \"UI: Cursor Set >> Busy|Idle\")"
        n120 = call <vilib>:"Add State(s) to Queue__jki_lib_state_machine.vi"("State(s) in (\"\")"=w286) -> ("States Out"=w281:string)  [unwired: 14 in]
        n121 = case shown="\"Idle\", Default" w282 {
          tunnel: w284 -> [w288 w290]
          tunnel: [w287 w289] -> w283
          frame "Idle", Default {
            n122 = call <vilib>:"Unset Busy.vi"("error in (no error)"=w288) -> ("error out"=w287:errorcluster)  [unwired: 10 in]
          }
          frame "Busy" {
            n123 = call <vilib>:"Set Busy.vi"("error in (no error)"=w290) -> ("error out"=w289:errorcluster)  [unwired: 9 in, 1 out]
          }
        }
      }
      frame "UI: Front Panel State" {
        # "Argument"
        # "Set Front Panel Open or Closed\n(Usage: \"UI: Front Panel State >> Open|Close\")"
        n124 = call <vilib>:"Add State(s) to Queue__jki_lib_state_machine.vi"("State(s) in (\"\")"=w297) -> ("States Out"=w291:string)  [unwired: 14 in]
        n125 = Unbundle By Name(w292) -> ("Core.Current VI Reference"=w294:refnum<vi>)
        n126 = case shown="\"Open\", Default" w293 {
          tunnel: w296 -> [w302 w314]
          tunnel: [w303 w315] -> w295
          tunnel: w294 -> [w298 w310]
          frame "Open", Default {
            n127 = property class="VI"(reference=w298, error in=w302) -> (reference out=w300:refnum<vi>, error out=w301:errorcluster, "Front Panel.Open"=w299:bool)
            n128 = case shown="False" w299 {
              tunnel: [w306 w309] -> w303
              tunnel: w301 -> [w305 w309]
              tunnel: w300 -> [w304 _]
              frame False {
                n129 = invoke class="VI" method="FP.Open"(reference=w304, error in=w305, "Activate"=TRUE, "State"=T4."Standard") -> (error out=w306:errorcluster)  [unwired: 1 in, 4 out]
              }
              frame True {
              }
            }
          }
          frame "Close" {
            n130 = property class="VI"(reference=w310, error in=w314) -> (reference out=w312:refnum<vi>, error out=w313:errorcluster, "Front Panel.Open"=w311:bool)
            n131 = case shown="True" w311 {
              tunnel: [w316 w319] -> w315
              tunnel: w313 -> [w316 w318]
              tunnel: w312 -> [_ w317]
              frame False {
              }
              frame True {
                n132 = invoke class="VI" method="FP.Close"(reference=w317, error in=w318) -> (error out=w319:errorcluster)  [unwired: 1 in, 2 out]
              }
            }
          }
        }
      }
      frame "---------- Macro ----------" {
        # "Do not put any code in this frame.\n(It is a separator no-op. You can make a copy of this frame to create a new Macro frame)"
        n133 = call <vilib>:"Add State(s) to Queue__jki_lib_state_machine.vi"("State(s) in (\"\")"=w323) -> ("States Out"=w320:string)  [unwired: 14 in]
      }
      frame "Macro: Initialize" {
        w325 = "Data: Initialize\nInitialize Core Data\nUI: Initialize\nUI: Front Panel State >> Open"  # Data: Initialize Initialize Core Data UI: Initialize UI: Front Panel State >> Open
        # "Initialization Macro\n(This is called once, when the VI starts)"
        n134 = call <vilib>:"Add State(s) to Queue__jki_lib_state_machine.vi"("State(s) in Front (\"\")"=w325, "State(s) in (\"\")"=w328) -> ("States Out"=w324:string)  [unwired: 13 in]
      }
      frame "Macro: Exit" {
        # "Exit Macro\n(This is called once, when the VI exits)"
        n135 = Unbundle By Name(w330) -> ("Core.Close Panel on Exit?"=w331:bool)
        n136 = Select(t="UI: Front Panel State >> Close", s=w331, f="") -> (s? t:f=w334:string)
        n137 = call <vilib>:"Add State(s) to Queue__jki_lib_state_machine.vi"("State(s) in (\"\")"=w334, "State(s) at Back (\"\")"="Data: Cleanup\nExit") -> ("States Out"=w332:string)  [unwired: 13 in]
        n138 = call <vilib>:"Add State(s) to Queue__jki_lib_state_machine.vi"("State(s) in Front (\"\")"=w332, "State(s) in (\"\")"=w338) -> ("States Out"=w329:string)  [unwired: 13 in]
      }
      frame "---------- New Category ----------" {
        n139 = call <vilib>:"Add State(s) to Queue__jki_lib_state_machine.vi"("State(s) in (\"\")"=w342) -> ("States Out"=w339:string)  [unwired: 14 in]
      }
      frame "Action: EMQ1Switch" {
        n140 = call <vilib>:"Add State(s) to Queue__jki_lib_state_machine.vi"("State(s) in (\"\")"=w352) -> ("States Out"=w351:string)  [unwired: 14 in]
        n141 = property on="CurrentSwitch limit" class="DigNum (strict)"() -> ("Value"=w347:dbl)  [unwired: 2 in, 2 out]
        n142 = property on="Current.Ch1::1" class="DigNum (strict)"() -> ("Value"=w348:dbl)  [unwired: 2 in, 2 out]
        n143 = Absolute Value(x=w348) -> (abs(x)=w350:dbl)
        n144 = Less?(x=w350, y=w347) -> (x < y?=w349:bool)
        n145 = case shown="True" w349 {
          tunnel: w346 -> [w354 w360]
          tunnel: [w354 w359] -> w345
          tunnel: w344 -> [w353 w358]
          tunnel: [w353 w355] -> w343
          frame False {
          }
          frame True {
            w357 = TRUE ("Value (Signaling)")
            w362 = FALSE ("Value (Signaling)")
            n146 = property on="DigitalOutput.Channel 0::4" class="Bool (strict)"(error in=w358, "Val(Sgnl)"=w357) -> (error out=w364:errorcluster)  [unwired: 1 in, 1 out]
            n147 = property on="SwitchWait" class="DigNum (strict)"() -> ("Value"=w361:dbl)  [unwired: 2 in, 2 out]
            n148 = call <userlib>:"Wait (ms)__ogtk.vi"("error in (no error)"=w364, "milliseconds to wait"=w361) -> ("error out"=w365:errorcluster)  [unwired: 8 in, 1 out]
            n149 = property on="DigitalOutput.Channel 0::4" class="Bool (strict)"(error in=w365, "Val(Sgnl)"=w362) -> (error out=w363:errorcluster)  [unwired: 1 in, 1 out]
            n150 = Bundle By Name(cluster=w360, "EMQ1PolaritySwitched"=w357) -> (w359:T5)
            n151 = property on="EMQ1Switch" class="Bool (strict)"(error in=w363, "Val(Sgnl)"=w362) -> (error out=w356:errorcluster)  [unwired: 1 in, 1 out]
            n152 = property on="EMQ1 indicator" class="Bool (strict)"(error in=w356, "Val(Sgnl)"=w357) -> (error out=w355:errorcluster)  [unwired: 1 in, 1 out]
          }
        }
      }
      frame "Action: EMQ1Reset" {
        n153 = call <vilib>:"Add State(s) to Queue__jki_lib_state_machine.vi"("State(s) in (\"\")"=w375) -> ("States Out"=w374:string)  [unwired: 14 in]
        n154 = property on="CurrentSwitch limit" class="DigNum (strict)"() -> ("Value"=w370:dbl)  [unwired: 2 in, 2 out]
        n155 = property on="Current.Ch1::1" class="DigNum (strict)"() -> ("Value"=w371:dbl)  [unwired: 2 in, 2 out]
        n156 = Absolute Value(x=w371) -> (abs(x)=w373:dbl)
        n157 = Less?(x=w373, y=w370) -> (x < y?=w372:bool)
        n158 = case shown="True" w372 {
          tunnel: w369 -> [w377 w383]
          tunnel: [w377 w382] -> w368
          tunnel: w367 -> [w376 w381]
          tunnel: [w376 w378] -> w366
          frame False {
          }
          frame True {
            w380 = FALSE ("Value (Signaling)")
            n159 = property on="DigitalOutput.Channel 1::4" class="Bool (strict)"(error in=w381, "Val(Sgnl)"=TRUE ("Value (Signaling)")) -> (error out=w387:errorcluster)  [unwired: 1 in, 1 out]
            n160 = property on="SwitchWait" class="DigNum (strict)"() -> ("Value"=w384:dbl)  [unwired: 2 in, 2 out]
            n161 = call <userlib>:"Wait (ms)__ogtk.vi"("error in (no error)"=w387, "milliseconds to wait"=w384) -> ("error out"=w388:errorcluster)  [unwired: 8 in, 1 out]
            n162 = property on="DigitalOutput.Channel 1::4" class="Bool (strict)"(error in=w388, "Val(Sgnl)"=w380) -> (error out=w385:errorcluster)  [unwired: 1 in, 1 out]
            n163 = Bundle By Name(cluster=w383, "EMQ1PolaritySwitched"=w380) -> (w382:T5)
            n164 = property on="EMQ1Reset" class="Bool (strict)"(error in=w385, "Val(Sgnl)"=w380) -> (error out=w379:errorcluster)  [unwired: 1 in, 1 out]
            n165 = property on="EMQ1 indicator" class="Bool (strict)"(error in=w379, "Val(Sgnl)"=w380) -> (error out=w378:errorcluster)  [unwired: 1 in, 1 out]
          }
        }
      }
      frame "Action: EMQ2Switch" {
        n166 = call <vilib>:"Add State(s) to Queue__jki_lib_state_machine.vi"("State(s) in (\"\")"=w398) -> ("States Out"=w397:string)  [unwired: 14 in]
        n167 = property on="CurrentSwitch limit" class="DigNum (strict)"() -> ("Value"=w393:dbl)  [unwired: 2 in, 2 out]
        n168 = property on="Current.Ch2::1" class="DigNum (strict)"() -> ("Value"=w394:dbl)  [unwired: 2 in, 2 out]
        n169 = Absolute Value(x=w394) -> (abs(x)=w396:dbl)
        n170 = Less?(x=w396, y=w393) -> (x < y?=w395:bool)
        n171 = case shown="True" w395 {
          tunnel: w392 -> [w400 w406]
          tunnel: [w400 w405] -> w391
          tunnel: w390 -> [w399 w404]
          tunnel: [w399 w401] -> w389
          frame False {
          }
          frame True {
            w403 = TRUE ("Value (Signaling)")
            w408 = FALSE ("Value (Signaling)")
            n172 = property on="DigitalOutput.Channel 2::4" class="Bool (strict)"(error in=w404, "Val(Sgnl)"=w403) -> (error out=w410:errorcluster)  [unwired: 1 in, 1 out]
            n173 = property on="SwitchWait" class="DigNum (strict)"() -> ("Value"=w407:dbl)  [unwired: 2 in, 2 out]
            n174 = call <userlib>:"Wait (ms)__ogtk.vi"("error in (no error)"=w410, "milliseconds to wait"=w407) -> ("error out"=w411:errorcluster)  [unwired: 8 in, 1 out]
            n175 = property on="DigitalOutput.Channel 2::4" class="Bool (strict)"(error in=w411, "Val(Sgnl)"=w408) -> (error out=w409:errorcluster)  [unwired: 1 in, 1 out]
            n176 = Bundle By Name(cluster=w406, "EMQ2PolaritySwitched"=w403) -> (w405:T5)
            n177 = property on="EMQ2Switch" class="Bool (strict)"(error in=w409, "Val(Sgnl)"=w408) -> (error out=w402:errorcluster)  [unwired: 1 in, 1 out]
            n178 = property on="EMQ2 indicator" class="Bool (strict)"(error in=w402, "Val(Sgnl)"=w403) -> (error out=w401:errorcluster)  [unwired: 1 in, 1 out]
          }
        }
      }
      frame "Action: EMQ2Reset" {
        n179 = call <vilib>:"Add State(s) to Queue__jki_lib_state_machine.vi"("State(s) in (\"\")"=w421) -> ("States Out"=w420:string)  [unwired: 14 in]
        n180 = property on="CurrentSwitch limit" class="DigNum (strict)"() -> ("Value"=w416:dbl)  [unwired: 2 in, 2 out]
        n181 = property on="Current.Ch2::1" class="DigNum (strict)"() -> ("Value"=w417:dbl)  [unwired: 2 in, 2 out]
        n182 = Absolute Value(x=w417) -> (abs(x)=w419:dbl)
        n183 = Less?(x=w419, y=w416) -> (x < y?=w418:bool)
        n184 = case shown="True" w418 {
          tunnel: w415 -> [w423 w429]
          tunnel: [w423 w428] -> w414
          tunnel: w413 -> [w422 w427]
          tunnel: [w422 w424] -> w412
          frame False {
          }
          frame True {
            w426 = FALSE ("Value (Signaling)")
            n185 = property on="DigitalOutput.Channel 3::4" class="Bool (strict)"(error in=w427, "Val(Sgnl)"=TRUE ("Value (Signaling)")) -> (error out=w433:errorcluster)  [unwired: 1 in, 1 out]
            n186 = property on="SwitchWait" class="DigNum (strict)"() -> ("Value"=w430:dbl)  [unwired: 2 in, 2 out]
            n187 = call <userlib>:"Wait (ms)__ogtk.vi"("error in (no error)"=w433, "milliseconds to wait"=w430) -> ("error out"=w434:errorcluster)  [unwired: 8 in, 1 out]
            n188 = property on="DigitalOutput.Channel 3::4" class="Bool (strict)"(error in=w434, "Val(Sgnl)"=w426) -> (error out=w431:errorcluster)  [unwired: 1 in, 1 out]
            n189 = Bundle By Name(cluster=w429, "EMQ2PolaritySwitched"=w426) -> (w428:T5)
            n190 = property on="EMQ2Reset" class="Bool (strict)"(error in=w431, "Val(Sgnl)"=w426) -> (error out=w425:errorcluster)  [unwired: 1 in, 1 out]
            n191 = property on="EMQ2 indicator" class="Bool (strict)"(error in=w425, "Val(Sgnl)"=w426) -> (error out=w424:errorcluster)  [unwired: 1 in, 1 out]
          }
        }
      }
      frame "Action: EMQ3Switch" {
        n192 = call <vilib>:"Add State(s) to Queue__jki_lib_state_machine.vi"("State(s) in (\"\")"=w444) -> ("States Out"=w443:string)  [unwired: 14 in]
        n193 = property on="CurrentSwitch limit" class="DigNum (strict)"() -> ("Value"=w439:dbl)  [unwired: 2 in, 2 out]
        n194 = property on="Current.Ch3::1" class="DigNum (strict)"() -> ("Value"=w440:dbl)  [unwired: 2 in, 2 out]
        n195 = Absolute Value(x=w440) -> (abs(x)=w442:dbl)
        n196 = Less?(x=w442, y=w439) -> (x < y?=w441:bool)
        n197 = case shown="True" w441 {
          tunnel: w438 -> [w446 w452]
          tunnel: [w446 w447] -> w437
          tunnel: w436 -> [w445 w451]
          tunnel: [w445 w450] -> w435
          frame False {
          }
          frame True {
            w449 = TRUE ("Value (Signaling)")
            w454 = FALSE ("Value (Signaling)")
            n198 = property on="DigitalOutput.Channel 4::4" class="Bool (strict)"(error in=w452, "Val(Sgnl)"=w449) -> (error out=w456:errorcluster)  [unwired: 1 in, 1 out]
            n199 = property on="SwitchWait" class="DigNum (strict)"() -> ("Value"=w453:dbl)  [unwired: 2 in, 2 out]
            n200 = call <userlib>:"Wait (ms)__ogtk.vi"("error in (no error)"=w456, "milliseconds to wait"=w453) -> ("error out"=w457:errorcluster)  [unwired: 8 in, 1 out]
            n201 = property on="DigitalOutput.Channel 4::4" class="Bool (strict)"(error in=w457, "Val(Sgnl)"=w454) -> (error out=w455:errorcluster)  [unwired: 1 in, 1 out]
            n202 = Bundle By Name(cluster=w451, "EMQ3PolaritySwitched"=w449) -> (w450:T5)
            n203 = property on="EMQ3Switch" class="Bool (strict)"(error in=w455, "Val(Sgnl)"=w454) -> (error out=w448:errorcluster)  [unwired: 1 in, 1 out]
            n204 = property on="EMQ3 indicator" class="Bool (strict)"(error in=w448, "Val(Sgnl)"=w449) -> (error out=w447:errorcluster)  [unwired: 1 in, 1 out]
          }
        }
      }
      frame "Action: EMQ3Reset" {
        n205 = call <vilib>:"Add State(s) to Queue__jki_lib_state_machine.vi"("State(s) in (\"\")"=w467) -> ("States Out"=w466:string)  [unwired: 14 in]
        n206 = property on="CurrentSwitch limit" class="DigNum (strict)"() -> ("Value"=w462:dbl)  [unwired: 2 in, 2 out]
        n207 = property on="Current.Ch3::1" class="DigNum (strict)"() -> ("Value"=w463:dbl)  [unwired: 2 in, 2 out]
        n208 = Absolute Value(x=w463) -> (abs(x)=w465:dbl)
        n209 = Less?(x=w465, y=w462) -> (x < y?=w464:bool)
        n210 = case shown="True" w464 {
          tunnel: w461 -> [w469 w475]
          tunnel: [w469 w470] -> w460
          tunnel: w459 -> [w468 w474]
          tunnel: [w468 w473] -> w458
          frame False {
          }
          frame True {
            w472 = FALSE ("Value (Signaling)")
            n211 = property on="DigitalOutput.Channel 5::4" class="Bool (strict)"(error in=w475, "Val(Sgnl)"=TRUE ("Value (Signaling)")) -> (error out=w479:errorcluster)  [unwired: 1 in, 1 out]
            n212 = property on="SwitchWait" class="DigNum (strict)"() -> ("Value"=w476:dbl)  [unwired: 2 in, 2 out]
            n213 = call <userlib>:"Wait (ms)__ogtk.vi"("error in (no error)"=w479, "milliseconds to wait"=w476) -> ("error out"=w480:errorcluster)  [unwired: 8 in, 1 out]
            n214 = property on="DigitalOutput.Channel 5::4" class="Bool (strict)"(error in=w480, "Val(Sgnl)"=w472) -> (error out=w477:errorcluster)  [unwired: 1 in, 1 out]
            n215 = Bundle By Name(cluster=w474, "EMQ3PolaritySwitched"=w472) -> (w473:T5)
            n216 = property on="EMQ3Reset" class="Bool (strict)"(error in=w477, "Val(Sgnl)"=w472) -> (error out=w471:errorcluster)  [unwired: 1 in, 1 out]
            n217 = property on="EMQ3 indicator" class="Bool (strict)"(error in=w471, "Val(Sgnl)"=w472) -> (error out=w470:errorcluster)  [unwired: 1 in, 1 out]
          }
        }
      }
      frame "Action: DegaussEMQ1" {
        n218 = Unbundle By Name(w484) -> ()  [unwired: 1 out]
        n219 = for {
          N: 700 -> [_]
          shift-right: [w490] -> w485
          shift-left: w486 -> [w489]
          n220 = call <vilib>:"Add State(s) to Queue__jki_lib_state_machine.vi"("State(s) in Front (\"\")"="Action: EMQ1DegaussCurrentCalculate\nAction: EMQ1DegaussCurrentApply" ("State(s) in Front (\"\")"), "State(s) in (\"\")"=w489) -> ("States Out"=w490:string)  [unwired: 13 in]
        }
        n221 = Bundle By Name(cluster=w484, "degauss loop"=0) -> (w483:T5)
      }
      frame "Action: DegaussEMQ2" {
        n222 = for {
          N: 700 -> [_]
          shift-right: [w500] -> w495
          shift-left: w496 -> [w499]
          n223 = call <vilib>:"Add State(s) to Queue__jki_lib_state_machine.vi"("State(s) in Front (\"\")"="Action: EMQ2DegaussCurrentCalculate\nAction: EMQ2DegaussCurrentApply" ("State(s) in Front (\"\")"), "State(s) in (\"\")"=w499) -> ("States Out"=w500:string)  [unwired: 13 in]
        }
        n224 = Bundle By Name(cluster=w494, "degauss loop"=0) -> (w493:T5)
      }
      frame "Action: DegaussEMQ3" {
        n225 = for {
          N: 700 -> [_]
          shift-right: [w510] -> w505
          shift-left: w506 -> [w509]
          n226 = call <vilib>:"Add State(s) to Queue__jki_lib_state_machine.vi"("State(s) in Front (\"\")"="Action: EMQ3DegaussCurrentCalculate\nAction: EMQ3DegaussCurrentApply" ("State(s) in Front (\"\")"), "State(s) in (\"\")"=w509) -> ("States Out"=w510:string)  [unwired: 13 in]
        }
        n227 = Bundle By Name(cluster=w504, "degauss loop"=0) -> (w503:T5)
      }
      frame "Action: EMQ1DegaussCurrentCalculate" {
        n228 = case shown="False" "abort1" {
          tunnel: w518 -> [w528 w578]
          tunnel: w517 -> [w534 _]
          tunnel: [w533 _] -> w516
          tunnel: [w529 w578] -> w515
          tunnel: w512 -> [w527 w577]
          tunnel: [w526 w577] -> w511
          frame False {
            n229 = Unbundle By Name(w528) -> ("EMQ1PolaritySwitched"=w525:bool)
            n230 = property on="Degauss max\ncurrent" class="DigNum (strict)"() -> ("Value"=w524:dbl)  [unwired: 2 in, 2 out]
            n231 = Unbundle By Name(w528) -> ("degauss loop"=w523:i32)
            n232 = property on="Current.Ch1::1" class="DigNum (strict)"() -> ("Value"=w522:dbl)  [unwired: 2 in, 2 out]
            n233 = call "CurrentCalculation.vi"("ReadBackCurrent"=w522, "iter"=w523, "daguas max current"=w524, "PolarityStatus"=w525) -> ("PositiveBool"=w519:bool, "SameSignBool"=w520:bool, "Setcurrent"=w521:dbl)  [unwired: 5 in]
            n234 = case shown="False" w520 {
              tunnel: w521 -> [w539 w575]
              tunnel: w534 -> [w541 w576]
              tunnel: [w540 w576] -> w533
              tunnel: [w538 w575] -> w532
              tunnel: w527 -> [w537 w574]
              tunnel: [w537 w574] -> w526
              tunnel: w519 -> [w536 _]
              frame False {
                n235 = case shown="False" w536 {
                  tunnel: w541 -> [w545 w560]
                  tunnel: [w548 w564] -> w540
                  tunnel: w539 -> [w546 w562]
                  tunnel: [w543 w561] -> w538
                  frame False {
                    n236 = property on="Current_Limit.Ch1::1" class="DigNum (strict)"("Val(Sgnl)"=0.0 ("Value (Signaling)")) -> ()  [unwired: 2 in, 2 out]
                    n237 = while {
                      tunnel: w546 -> [w551]
                      tunnel: [w550] -> w543
                      tunnel: w545 -> [w549]
                      tunnel: [w549] -> w544
                      stop <- w553 stop-if-true
                      n238 = Wait (ms)(milliseconds to wait=u32 100) -> ()  [unwired: 1 out]
                      n239 = Absolute Value(x=w551) -> (abs(x)=w550:dbl)
                      n240 = property on="Current.Ch1::1" class="DigNum (strict)"() -> ("Value"=w556:dbl)  [unwired: 2 in, 2 out]
                      n241 = Absolute Value(x=w556) -> (abs(x)=w557:dbl)
                      n242 = Subtract(x=w557, y=w550) -> (x-y=w555:dbl)
                      n243 = Less?(x=w555, y=0.02) -> (x < y?=w553:bool)
                    }
                    n244 = call <vilib>:"Add State(s) to Queue__jki_lib_state_machine.vi"("State(s) in Front (\"\")"="Action: EMQ1Switch" ("State(s) in Front (\"\")"), "State(s) in (\"\")"=w544) -> ("States Out"=w548:string)  [unwired: 13 in]
                  }
                  frame True {
                    n245 = property on="Current_Limit.Ch1::1" class="DigNum (strict)"("Val(Sgnl)"=0.0 ("Value (Signaling)")) -> ()  [unwired: 2 in, 2 out]
                    n246 = while {
                      tunnel: w562 -> [w567]
                      tunnel: [w566] -> w561
                      tunnel: w560 -> [w565]
                      tunnel: [w565] -> w559
                      stop <- w569 stop-if-true
                      n247 = Wait (ms)(milliseconds to wait=u32 100) -> ()  [unwired: 1 out]
                      n248 = Absolute Value(x=w567) -> (abs(x)=w566:dbl)
                      n249 = property on="Current.Ch1::1" class="DigNum (strict)"() -> ("Value"=w572:dbl)  [unwired: 2 in, 2 out]
                      n250 = Absolute Value(x=w572) -> (abs(x)=w573:dbl)
                      n251 = Subtract(x=w573, y=w566) -> (x-y=w571:dbl)
                      n252 = Less?(x=w571, y=0.02) -> (x < y?=w569:bool)
                    }
                    n253 = call <vilib>:"Add State(s) to Queue__jki_lib_state_machine.vi"("State(s) in Front (\"\")"="Action: EMQ1Reset" ("State(s) in Front (\"\")"), "State(s) in (\"\")"=w559) -> ("States Out"=w564:string)  [unwired: 13 in]
                  }
                }
              }
              frame True {
              }
            }
            n254 = Increment(x=w523) -> (x+1=w535:i32)
            n255 = Bundle By Name(cluster=w528, "degauss loop"=w535) -> (w530:T5)
            n256 = Absolute Value(x=w532) -> (abs(x)=w531:dbl)
            n257 = Bundle By Name(cluster=w530, "EMQ1DegaussSetCur"=w531) -> (w529:T5)
          }
          frame True {
          }
        }
        n258 = Wait (ms)(milliseconds to wait=u32 500) -> ()  [unwired: 1 out]
      }
      frame "Action: EMQ2DegaussCurrentCalculate" {
        n259 = case shown="False" "abort2" {
          tunnel: w586 -> [w596 w646]
          tunnel: w585 -> [w602 _]
          tunnel: [w601 _] -> w584
          tunnel: [w597 w646] -> w583
          tunnel: w580 -> [w595 w645]
          tunnel: [w594 w645] -> w579
          frame False {
            n260 = Unbundle By Name(w596) -> ("EMQ2PolaritySwitched"=w593:bool)
            n261 = property on="Degauss max\ncurrent" class="DigNum (strict)"() -> ("Value"=w592:dbl)  [unwired: 2 in, 2 out]
            n262 = Unbundle By Name(w596) -> ("degauss loop"=w591:i32)
            n263 = property on="Current.Ch2::1" class="DigNum (strict)"() -> ("Value"=w590:dbl)  [unwired: 2 in, 2 out]
            n264 = call "CurrentCalculation.vi"("ReadBackCurrent"=w590, "iter"=w591, "daguas max current"=w592, "PolarityStatus"=w593) -> ("PositiveBool"=w587:bool, "SameSignBool"=w588:bool, "Setcurrent"=w589:dbl)  [unwired: 5 in]
            n265 = case shown="False" w588 {
              tunnel: w589 -> [w607 w643]
              tunnel: w602 -> [w609 w644]
              tunnel: [w608 w644] -> w601
              tunnel: [w606 w643] -> w600
              tunnel: w595 -> [w605 w642]
              tunnel: [w605 w642] -> w594
              tunnel: w587 -> [w604 _]
              frame False {
                n266 = case shown="True" w604 {
                  tunnel: w609 -> [w613 w628]
                  tunnel: [w616 w632] -> w608
                  tunnel: w607 -> [w614 w630]
                  tunnel: [w611 w629] -> w606
                  frame False {
                    n267 = property on="Current_Limit.Ch2::1" class="DigNum (strict)"("Val(Sgnl)"=0.0 ("Value (Signaling)")) -> ()  [unwired: 2 in, 2 out]
                    n268 = while {
                      tunnel: w614 -> [w619]
                      tunnel: [w618] -> w611
                      tunnel: w613 -> [w617]
                      tunnel: [w617] -> w612
                      stop <- w621 stop-if-true
                      n269 = Wait (ms)(milliseconds to wait=u32 100) -> ()  [unwired: 1 out]
                      n270 = Absolute Value(x=w619) -> (abs(x)=w618:dbl)
                      n271 = property on="Current.Ch2::1" class="DigNum (strict)"() -> ("Value"=w624:dbl)  [unwired: 2 in, 2 out]
                      n272 = Absolute Value(x=w624) -> (abs(x)=w625:dbl)
                      n273 = Subtract(x=w625, y=w618) -> (x-y=w623:dbl)
                      n274 = Less?(x=w623, y=0.02) -> (x < y?=w621:bool)
                    }
                    n275 = call <vilib>:"Add State(s) to Queue__jki_lib_state_machine.vi"("State(s) in Front (\"\")"="Action: EMQ2Switch" ("State(s) in Front (\"\")"), "State(s) in (\"\")"=w612) -> ("States Out"=w616:string)  [unwired: 13 in]
                  }
                  frame True {
                    n276 = property on="Current_Limit.Ch2::1" class="DigNum (strict)"("Val(Sgnl)"=0.0 ("Value (Signaling)")) -> ()  [unwired: 2 in, 2 out]
                    n277 = while {
                      tunnel: w630 -> [w635]
                      tunnel: [w634] -> w629
                      tunnel: w628 -> [w633]
                      tunnel: [w633] -> w627
                      stop <- w637 stop-if-true
                      n278 = Wait (ms)(milliseconds to wait=u32 100) -> ()  [unwired: 1 out]
                      n279 = Absolute Value(x=w635) -> (abs(x)=w634:dbl)
                      n280 = property on="Current.Ch2::1" class="DigNum (strict)"() -> ("Value"=w640:dbl)  [unwired: 2 in, 2 out]
                      n281 = Absolute Value(x=w640) -> (abs(x)=w641:dbl)
                      n282 = Subtract(x=w641, y=w634) -> (x-y=w639:dbl)
                      n283 = Less?(x=w639, y=0.02) -> (x < y?=w637:bool)
                    }
                    n284 = call <vilib>:"Add State(s) to Queue__jki_lib_state_machine.vi"("State(s) in Front (\"\")"="Action: EMQ2Reset" ("State(s) in Front (\"\")"), "State(s) in (\"\")"=w627) -> ("States Out"=w632:string)  [unwired: 13 in]
                  }
                }
              }
              frame True {
              }
            }
            n285 = Increment(x=w591) -> (x+1=w603:i32)
            n286 = Bundle By Name(cluster=w596, "degauss loop"=w603) -> (w598:T5)
            n287 = Absolute Value(x=w600) -> (abs(x)=w599:dbl)
            n288 = Bundle By Name(cluster=w598, "EMQ2DegaussSetCur"=w599) -> (w597:T5)
          }
          frame True {
          }
        }
        n289 = Wait (ms)(milliseconds to wait=u32 500) -> ()  [unwired: 1 out]
      }
      frame "Action: EMQ3DegaussCurrentCalculate" {
        n290 = case shown="False" "abort3" {
          tunnel: w654 -> [w664 w714]
          tunnel: w653 -> [w670 _]
          tunnel: [w669 _] -> w652
          tunnel: [w665 w714] -> w651
          tunnel: w648 -> [w663 w713]
          tunnel: [w662 w713] -> w647
          frame False {
            n291 = Unbundle By Name(w664) -> ("EMQ3PolaritySwitched"=w661:bool)
            n292 = property on="Degauss max\ncurrent" class="DigNum (strict)"() -> ("Value"=w660:dbl)  [unwired: 2 in, 2 out]
            n293 = Unbundle By Name(w664) -> ("degauss loop"=w659:i32)
            n294 = property on="Current.Ch3::1" class="DigNum (strict)"() -> ("Value"=w658:dbl)  [unwired: 2 in, 2 out]
            n295 = call "CurrentCalculation.vi"("ReadBackCurrent"=w658, "iter"=w659, "daguas max current"=w660, "PolarityStatus"=w661) -> ("PositiveBool"=w655:bool, "SameSignBool"=w656:bool, "Setcurrent"=w657:dbl)  [unwired: 5 in]
            n296 = case shown="False" w656 {
              tunnel: w657 -> [w675 w711]
              tunnel: w670 -> [w677 w712]
              tunnel: [w676 w712] -> w669
              tunnel: [w674 w711] -> w668
              tunnel: w663 -> [w673 w710]
              tunnel: [w673 w710] -> w662
              tunnel: w655 -> [w672 _]
              frame False {
                n297 = case shown="True" w672 {
                  tunnel: w677 -> [w681 w696]
                  tunnel: [w684 w700] -> w676
                  tunnel: w675 -> [w682 w698]
                  tunnel: [w679 w697] -> w674
                  frame False {
                    n298 = property on="Current_Limit.Ch3::1" class="DigNum (strict)"("Val(Sgnl)"=0.0 ("Value (Signaling)")) -> ()  [unwired: 2 in, 2 out]
                    n299 = while {
                      tunnel: w682 -> [w687]
                      tunnel: [w686] -> w679
                      tunnel: w681 -> [w685]
                      tunnel: [w685] -> w680
                      stop <- w689 stop-if-true
                      n300 = Wait (ms)(milliseconds to wait=u32 100) -> ()  [unwired: 1 out]
                      n301 = Absolute Value(x=w687) -> (abs(x)=w686:dbl)
                      n302 = property on="Current.Ch3::1" class="DigNum (strict)"() -> ("Value"=w692:dbl)  [unwired: 2 in, 2 out]
                      n303 = Absolute Value(x=w692) -> (abs(x)=w693:dbl)
                      n304 = Subtract(x=w693, y=w686) -> (x-y=w691:dbl)
                      n305 = Less?(x=w691, y=0.02) -> (x < y?=w689:bool)
                    }
                    n306 = call <vilib>:"Add State(s) to Queue__jki_lib_state_machine.vi"("State(s) in Front (\"\")"="Action: EMQ3Switch" ("State(s) in Front (\"\")"), "State(s) in (\"\")"=w680) -> ("States Out"=w684:string)  [unwired: 13 in]
                  }
                  frame True {
                    n307 = property on="Current_Limit.Ch3::1" class="DigNum (strict)"("Val(Sgnl)"=0.0 ("Value (Signaling)")) -> ()  [unwired: 2 in, 2 out]
                    n308 = while {
                      tunnel: w698 -> [w703]
                      tunnel: [w702] -> w697
                      tunnel: w696 -> [w701]
                      tunnel: [w701] -> w695
                      stop <- w705 stop-if-true
                      n309 = Wait (ms)(milliseconds to wait=u32 100) -> ()  [unwired: 1 out]
                      n310 = Absolute Value(x=w703) -> (abs(x)=w702:dbl)
                      n311 = property on="Current.Ch3::1" class="DigNum (strict)"() -> ("Value"=w708:dbl)  [unwired: 2 in, 2 out]
                      n312 = Absolute Value(x=w708) -> (abs(x)=w709:dbl)
                      n313 = Subtract(x=w709, y=w702) -> (x-y=w707:dbl)
                      n314 = Less?(x=w707, y=0.02) -> (x < y?=w705:bool)
                    }
                    n315 = call <vilib>:"Add State(s) to Queue__jki_lib_state_machine.vi"("State(s) in Front (\"\")"="Action: EMQ3Reset" ("State(s) in Front (\"\")"), "State(s) in (\"\")"=w695) -> ("States Out"=w700:string)  [unwired: 13 in]
                  }
                }
              }
              frame True {
              }
            }
            n316 = Increment(x=w659) -> (x+1=w671:i32)
            n317 = Bundle By Name(cluster=w664, "degauss loop"=w671) -> (w666:T5)
            n318 = Absolute Value(x=w668) -> (abs(x)=w667:dbl)
            n319 = Bundle By Name(cluster=w666, "EMQ3DegaussSetCur"=w667) -> (w665:T5)
          }
          frame True {
          }
        }
        n320 = Wait (ms)(milliseconds to wait=u32 500) -> ()  [unwired: 1 out]
      }
      frame "Action: EMQ1DegaussCurrentApply" {
        n321 = Unbundle By Name(w720) -> ("EMQ1DegaussSetCur"=w717:dbl)
        n322 = property on="Current_Limit.Ch1::1" class="DigNum (strict)"("Val(Sgnl)"=w717) -> ()  [unwired: 2 in, 2 out]
        n323 = while {
          tunnel: w717 -> [w728]
          tunnel: w716 -> [w722]
          tunnel: [w722] -> w715
          stop <- w724 stop-if-true
          n324 = Wait (ms)(milliseconds to wait=u32 100) -> ()  [unwired: 1 out]
          n325 = property on="Current.Ch1::1" class="DigNum (strict)"() -> ("Value"=w729:dbl)  [unwired: 2 in, 2 out]
          n326 = Absolute Value(x=w729) -> (abs(x)=w730:dbl)
          n327 = Absolute Value(x=w728) -> (abs(x)=w727:dbl)
          n328 = Subtract(x=w730, y=w727) -> (x-y=w726:dbl)
          n329 = Less?(x=w726, y=0.02) -> (x < y?=w724:bool)
        }
        n330 = call <vilib>:"Add State(s) to Queue__jki_lib_state_machine.vi"("State(s) in Front (\"\")"="MakeChart" ("State(s) in Front (\"\")"), "State(s) in (\"\")"=w715) -> ("States Out"=w718:string)  [unwired: 13 in]
      }
      frame "Action: EMQ2DegaussCurrentApply" {
        n331 = Unbundle By Name(w736) -> ("EMQ2DegaussSetCur"=w731:dbl)
        n332 = property on="Current_Limit.Ch2::1" class="DigNum (strict)"("Val(Sgnl)"=w731) -> ()  [unwired: 2 in, 2 out]
        n333 = while {
          tunnel: w731 -> [w744]
          tunnel: w733 -> [w738]
          tunnel: [w738] -> w732
          stop <- w740 stop-if-true
          n334 = Wait (ms)(milliseconds to wait=u32 100) -> ()  [unwired: 1 out]
          n335 = property on="Current.Ch2::1" class="DigNum (strict)"() -> ("Value"=w745:dbl)  [unwired: 2 in, 2 out]
          n336 = Absolute Value(x=w745) -> (abs(x)=w746:dbl)
          n337 = Absolute Value(x=w744) -> (abs(x)=w743:dbl)
          n338 = Subtract(x=w746, y=w743) -> (x-y=w742:dbl)
          n339 = Less?(x=w742, y=0.02) -> (x < y?=w740:bool)
        }
        n340 = call <vilib>:"Add State(s) to Queue__jki_lib_state_machine.vi"("State(s) in Front (\"\")"="MakeChart" ("State(s) in Front (\"\")"), "State(s) in (\"\")"=w732) -> ("States Out"=w734:string)  [unwired: 13 in]
      }
      frame "Action: EMQ3DegaussCurrentApply" {
        n341 = Unbundle By Name(w752) -> ("EMQ3DegaussSetCur"=w747:dbl)
        n342 = property on="Current_Limit.Ch3::1" class="DigNum (strict)"("Val(Sgnl)"=w747) -> ()  [unwired: 2 in, 2 out]
        n343 = while {
          tunnel: w747 -> [w760]
          tunnel: w749 -> [w754]
          tunnel: [w754] -> w748
          stop <- w756 stop-if-true
          n344 = Wait (ms)(milliseconds to wait=u32 100) -> ()  [unwired: 1 out]
          n345 = property on="Current.Ch3::1" class="DigNum (strict)"() -> ("Value"=w761:dbl)  [unwired: 2 in, 2 out]
          n346 = Absolute Value(x=w761) -> (abs(x)=w762:dbl)
          n347 = Absolute Value(x=w760) -> (abs(x)=w759:dbl)
          n348 = Subtract(x=w762, y=w759) -> (x-y=w758:dbl)
          n349 = Less?(x=w758, y=0.02) -> (x < y?=w756:bool)
        }
        n350 = call <vilib>:"Add State(s) to Queue__jki_lib_state_machine.vi"("State(s) in Front (\"\")"="MakeChart" ("State(s) in Front (\"\")"), "State(s) in (\"\")"=w748) -> ("States Out"=w750:string)  [unwired: 13 in]
      }
      frame "MakeChart" {
        n351 = Unbundle By Name(w767) -> ("EMQ1PolaritySwitched"=w773:bool)
        n352 = Unbundle By Name(w767) -> ("EMQ2PolaritySwitched"=w776:bool)
        n353 = Unbundle By Name(w767) -> ("EMQ3PolaritySwitched"=w770:bool)
        n354 = property on="Current.Ch3::1" class="DigNum (strict)"() -> ("Value"=w769:dbl)  [unwired: 2 in, 2 out]
        n355 = case shown="True" w773 {
          tunnel: [1 -1] -> w771
          frame False {
          }
          frame True {
          }
        }
        n356 = case shown="False" w776 {
          tunnel: [1 -1] -> w775
          frame False {
          }
          frame True {
          }
        }
        n357 = case shown="False" w770 {
          tunnel: [1 -1] -> w768
          frame False {
          }
          frame True {
          }
        }
        n358 = property on="Current.Ch1::1" class="DigNum (strict)"() -> ("Value"=w772:dbl)  [unwired: 2 in, 2 out]
        n359 = property on="Current.Ch2::1" class="DigNum (strict)"() -> ("Value"=w774:dbl)  [unwired: 2 in, 2 out]
        n360 = Multiply(x=w774, y=w775) -> (x*y=w765:dbl)
        n361 = Multiply(x=w769, y=w768) -> (x*y=w764:dbl)
        n362 = Multiply(x=w772, y=w771) -> (x*y=w766:dbl)
        n363 = Bundle(w766, w765, w764) -> (→"Chart":cluster{dbl, dbl, dbl})  [unwired: 1 in]
      }
    }
  }
  n364 = disable-structure shown="Disabled" {
    frame Disabled {
      n365 = Wait (ms)(milliseconds to wait=u32 100) -> ()  [unwired: 1 out]
      n366 = property on="Current_Limit.Ch1::1" class="DigNum (strict)"("Val(Sgnl)"=0.0 ("Value (Signaling)")) -> ()  [unwired: 2 in, 2 out]
      n367 = Wait (ms)(milliseconds to wait=u32 100) -> ()  [unwired: 1 out]
      n368 = property on="Current_Limit.Ch1::1" class="DigNum (strict)"("Val(Sgnl)"=0.0 ("Value (Signaling)")) -> ()  [unwired: 2 in, 2 out]
    }
    frame Enabled {
    }
  }
